vi "ExtractLastArmpressureAsActivity.vi"(9 "Activity":dbl[](array[numeric]), 11 "Non-activity":dbl[](array[numeric])) -> (1 "Activity":dbl[](array[numeric]), 3 "Non-activity":dbl[](array[numeric]))   [LabVIEW 2013, in "main.lvlib"]
uses:
  main.lvlib
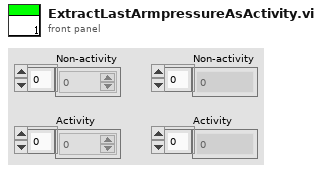
[diagram p1: front panel]
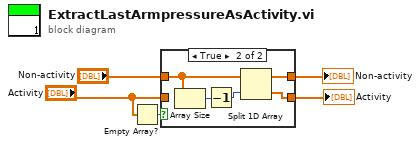
[diagram p0: block diagram]
diagram:
  n1 = Empty Array?(array="Activity") -> (empty?=w1:bool)
  n2 = case shown="True" w1 {
    tunnel: "Non-activity" -> [w6 w10]
    tunnel: "Activity" -> [w7 _]
    tunnel: [w7 w11] -> w4
    tunnel: [w6 w12] -> w5
    frame False {
    }
    frame True {
      n3 = Array Size(array=w10) -> (size(s)=w9:i32)
      n4 = Decrement(x=w9) -> (x-1=w8:i32)
      n5 = Split 1D Array(array=w10, index=w8) -> (first subarray=w12:dbl[], second subarray=w11:dbl[])
    }
  }
  "Non-activity" <- w5
  "Activity" <- w4
